vi "reservation tests.vi"() -> ()   [LabVIEW 2016]
uses:
  Resource Reservation DB/Resource Reservation DB.lvclass
  Resource Reservation DB/resrouce type.ctl
panel:
  out "Reserver":string
  out "index":i32
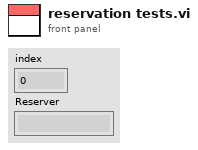
[diagram p1: front panel]
types:
  T1 = typedef "FPGA Addon Shared.lvlib/Resource Reservation DB.lvclass/resrouce type.ctl" = enum16{"Scalar Input", "Scalar Output", "Waveform Input", "Waveform Output"}
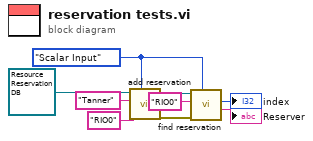
[diagram p0: block diagram]
diagram:
  w3 = resrouce_type."Scalar Input" ("Resource Type")
  n1 = call "add reservation.vi"("Resource Type"=w3, "Name in Bitfile"="RIO0", "Reserver"="Tanner", "Resource Reservation DB in"=refnum<class "Resource Reservation DB.lvclass"> refnum) -> ("error out"=w4:errorcluster, "Resource Reservation DB out"=w6:refnum<class "Resource Reservation DB.lvclass">)  [unwired: 6 in]
  n2 = call "find reservation.vi"("Resource Type"=w3, "error in (no error)"=w4, "Name in Bitfile"="RIO0", "Resource Reservation DB in"=w6) -> ("Reserver"=→"Reserver":string, "index"=→"index":i32)  [unwired: 4 in, 2 out]
